vi "DiffY.vi"(2 "Array in":dbl[][](array[numeric]), 3 "DiffY":bool caption="Scan") -> (0 "Array out":dbl[][](array[numeric]))   [LabVIEW 2018]
uses:
  <vilib>/Analysis/NI_AALPro.lvlib
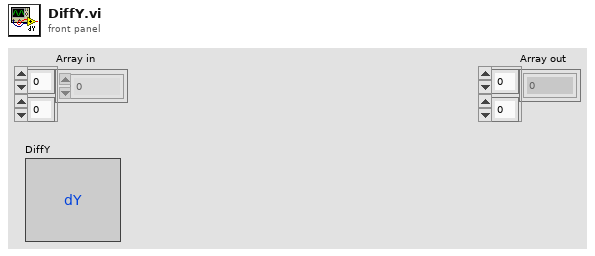
[diagram p1: front panel]
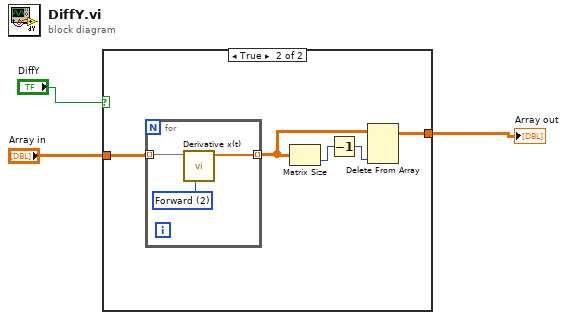
[diagram p0: block diagram]
diagram:
  n1 = case shown="True" "DiffY" {
    tunnel: [w4 w6] -> w1
    tunnel: "Array in" -> [w4 w5]
    frame False {
    }
    frame True {
      n2 = for {
        tunnel: w5 -> [w12] mode=indexing
        tunnel: [w10] -> w8 mode=indexing
        w11 = u16 2 items=["2nd Order Central", "4th Order Central", "Forward", "Backward"] ("method")
        n3 = call <vilib>:"Derivative x(t).vi"("method"=w11, "X"=w12) -> ("dX/dt"=w10:dbl[])  [unwired: 8 in, 1 out]
      }
      n4 = Matrix Size(0:w8) -> (2:w7:i32)  [unwired: 1 out]
      n5 = Decrement(x=w7) -> (x-1=w9:i32)
      n6 = Delete From Array(array=w8, index (col)=w9) -> (array with subset deleted=w6:dbl[][])  [unwired: 2 in, 1 out]
    }
  }
  "Array out" <- w1
